vi "Balance.vi"() -> ()   [LabVIEW 2013, in "ToplevelControllerLibrary.lvlib"]
uses:
  ToplevelControllerLibrary.lvlib
panel:
  out "error out":errorcluster
  in  "error in (no error)":errorcluster
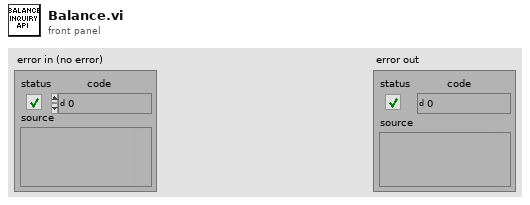
[diagram p1: front panel]
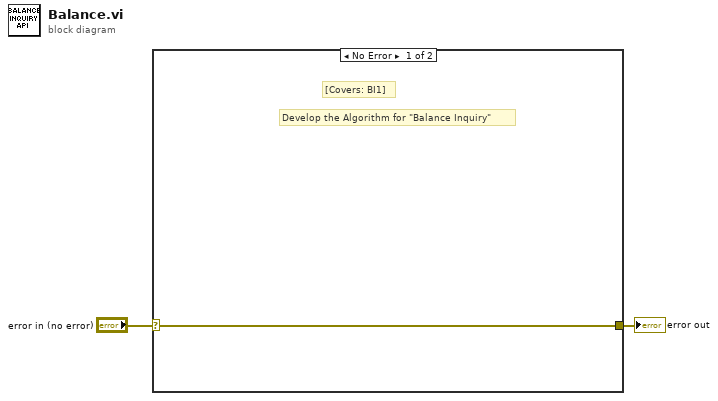
[diagram p0: block diagram]
diagram:
  n1 = case shown="No Error" "error in (no error)" {
    selector: "error in (no error)" -> [w3 w4]
    tunnel: [w3 w4] -> w1
    frame No Error {
      # "[Covers: BI1]"
      # "Develop the Algorithm for \"Balance Inquiry\""
    }
    frame Error {
    }
  }
  "error out" <- w1
